vi "Асинхронный ввод для PMT.vi"() -> ()   [LabVIEW 2016]
panel:
  out "Module name":string
  in  "stop":bool
  out "Канал АЦП 2":dbl(knob) scale=-10.0..10.0 scale format="%.1f"
  out "Канал АЦП 1":dbl(knob) scale=-10.0..10.0 scale format="%.1f"
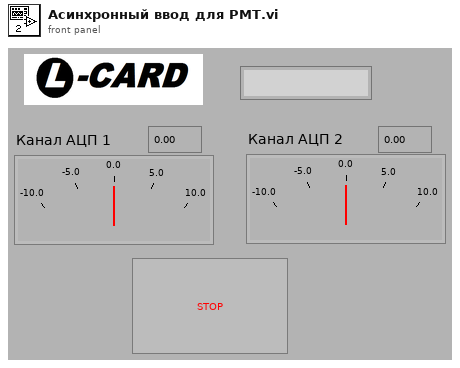
[diagram p1: front panel]
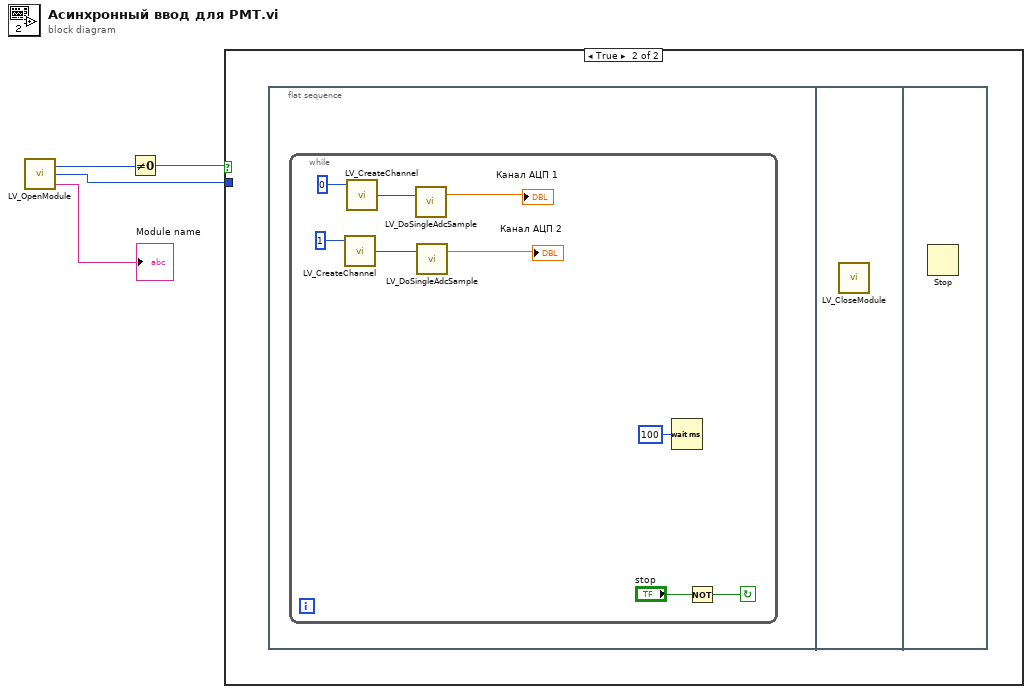
[diagram p0: block diagram]
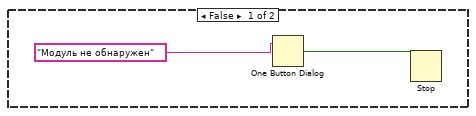
[diagram p2: hidden frame]
diagram:
  n1 = call "LV_OpenModule.vi"() -> ("Module Name"=→"Module name":string, "Module id"=w2:u8, "Error"=w3:u8)
  n2 = Not Equal To 0?(x=w3) -> (x != 0?=w4:bool)
  n3 = case shown="True" w4 {
    tunnel: w2 -> [_ _]
    frame False {
      n4 = One Button Dialog(message="Модуль не обнаружен") -> (true=w5:bool)  [unwired: 1 in]
      n5 = Stop(stop? (T)=w5) -> ()
    }
    frame True {
      n6 = flat-sequence {
        frame #0 {
          n7 = while {
            stop <- w14 continue-if-true
            n8 = stacked-sequence {
              frame #0 {
              }
              frame #1 {
              }
            }
            n9 = call "LV_CreateChannel.vi"("Channel"=u16 1) -> ("Logical channel"=w9:u16)  [unwired: 2 in]
            n10 = call "LV_CreateChannel.vi"("Channel"=u16 0) -> ("Logical channel"=w11:u16)  [unwired: 2 in]
            n11 = call "LV_DoSingleAdcSample.vi"("Logical ch Num"=w11) -> ("Result"=→"Канал АЦП 1":dbl)  [unwired: 1 in, 1 out]
            n12 = call "LV_DoSingleAdcSample.vi"("Logical ch Num"=w9) -> ("Result"=→"Канал АЦП 2":dbl)  [unwired: 1 in, 1 out]
            n13 = Wait (ms)(milliseconds to wait=u32 100) -> ()  [unwired: 1 out]
            n14 = Not(x="stop") -> (.not. x?=w14:bool)
          }
        }
        frame #1 {
          n15 = call "LV_CloseModule.vi"() -> ()  [unwired: 1 in]
        }
        frame #2 {
          n16 = Stop() -> ()  [unwired: 1 in]
        }
      }
    }
  }
